vi "Read channel name (_CHANNEL1_).vi"(8 "error in (no error)":errorcluster, 11 "Configure Channel Msg in":refnum<class "Configure Channel Msg.lvclass">) -> (0 "error out":errorcluster, 2 "channel name (\"CHANNEL1\")":string="CHANNEL1", 3 "Configure Channel Msg out":refnum<class "Configure Channel Msg.lvclass">)   [LabVIEW 2015, in "CS++Scope.lvlib" / "Configure Channel Msg.lvclass"]
uses:
  Configure Channel Msg.lvclass
  Configure Channel Msg.lvclass/Configure Channel Msg.ctl
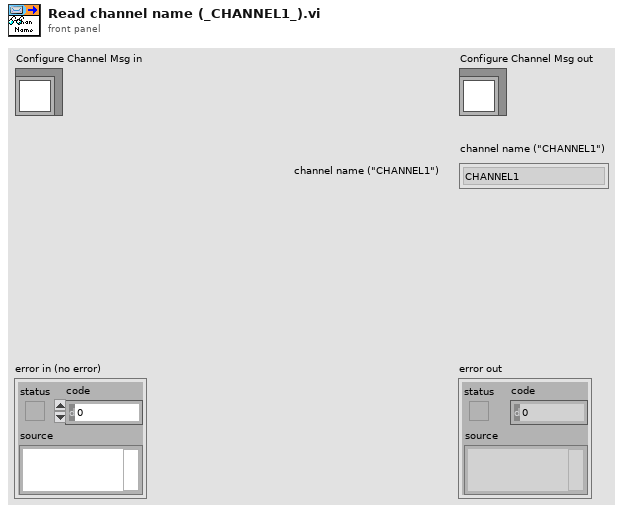
[diagram p1: front panel]
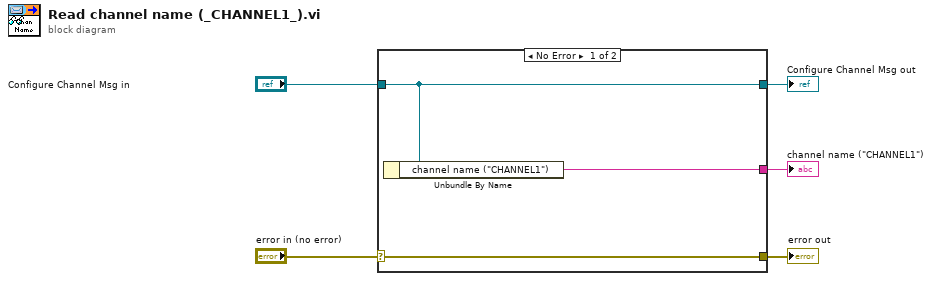
[diagram p0: block diagram]
diagram:
  n1 = case shown="No Error" "error in (no error)" {
    selector: "error in (no error)" -> [w8 w9]
    tunnel: [w8 w9] -> w4
    tunnel: [w7 w10] -> w2
    tunnel: "Configure Channel Msg in" -> [w7 w10]
    tunnel: [w6 _] -> w1
    frame No Error {
      n2 = Unbundle By Name(w7) -> ("channel name (\"CHANNEL1\")"=w6:string)
    }
    frame Error {
    }
  }
  "error out" <- w4
  "Configure Channel Msg out" <- w2
  "channel name (\"CHANNEL1\")" <- w1
